vi "Fgen Basic Standard Function.vi"() -> ()   [LabVIEW 2015]
doc: "This example shows how to use Standard Function mode. This is a basic example that shows the smallest amount of code necessary to generate a standard waveform."
uses:
  <instrlib>/niFgen/niFgen.llb/niFgen Output Mode.ctl
panel:
  in  "持续时间":dbl
  in  "DC Offset":dbl format="%.4f"
  in  "Standard Waveform":u16(ring) items=["Sine", "Square", "Triangle", "Ramp Up", "Ramp Down", "DC", "Noise"]
  in  "FGEN Resource Name":refnum<k15>
  in  "Frequency":dbl=1000000.0 format="%.2p"
  in  "Amplitude":dbl=2.0 format="%0_3g"
  # "Overview: Demonstrates how to configure an NI Signal Source to generate a basic standard function.\nSoftware Requirements: NI-FGEN\nHardware Requirements: PXI-5401, PCI-5401, PXI-5402, PCI-5402, PXI-5406, PCI-5406, PXI-5411, PCI-5411, AT-5411, PXI-5412, PCI-5412, PXIe-5413, PXI-5421, PCI-5421, PXI-5422, PXIe-5423, PXI-5431, PCI-5431, PXIe-5433, PXI-5441, NI PXIe-5442, NI PXIe-5450, or NI PXIe-5451 \nInstructions:\n1. Select the FGEN Resource Name as configured in the Measurement & Automation Explorer.\n2. Select the Standard Waveform to be generated.\n3. Specify the desired Frequency for the waveform.\n4. Select to Amplitude of the waveform.\n5. Run the VI.\n6. Click Stop to stop the VI."
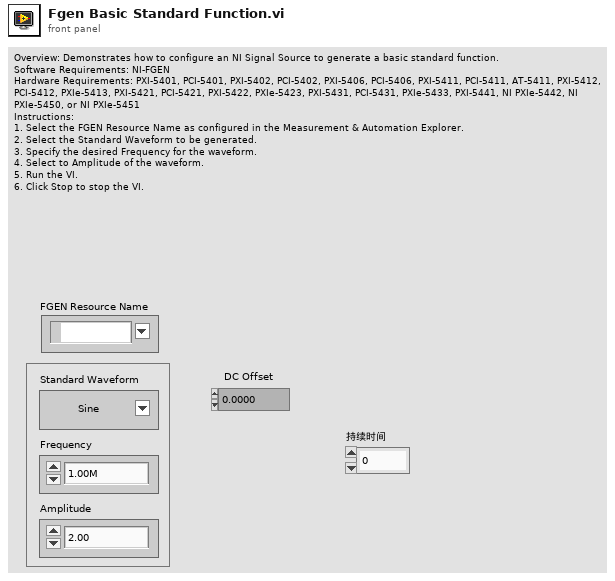
[diagram p1: front panel]
types:
  T1 = typedef "niFgen Output Mode.ctl" = u32
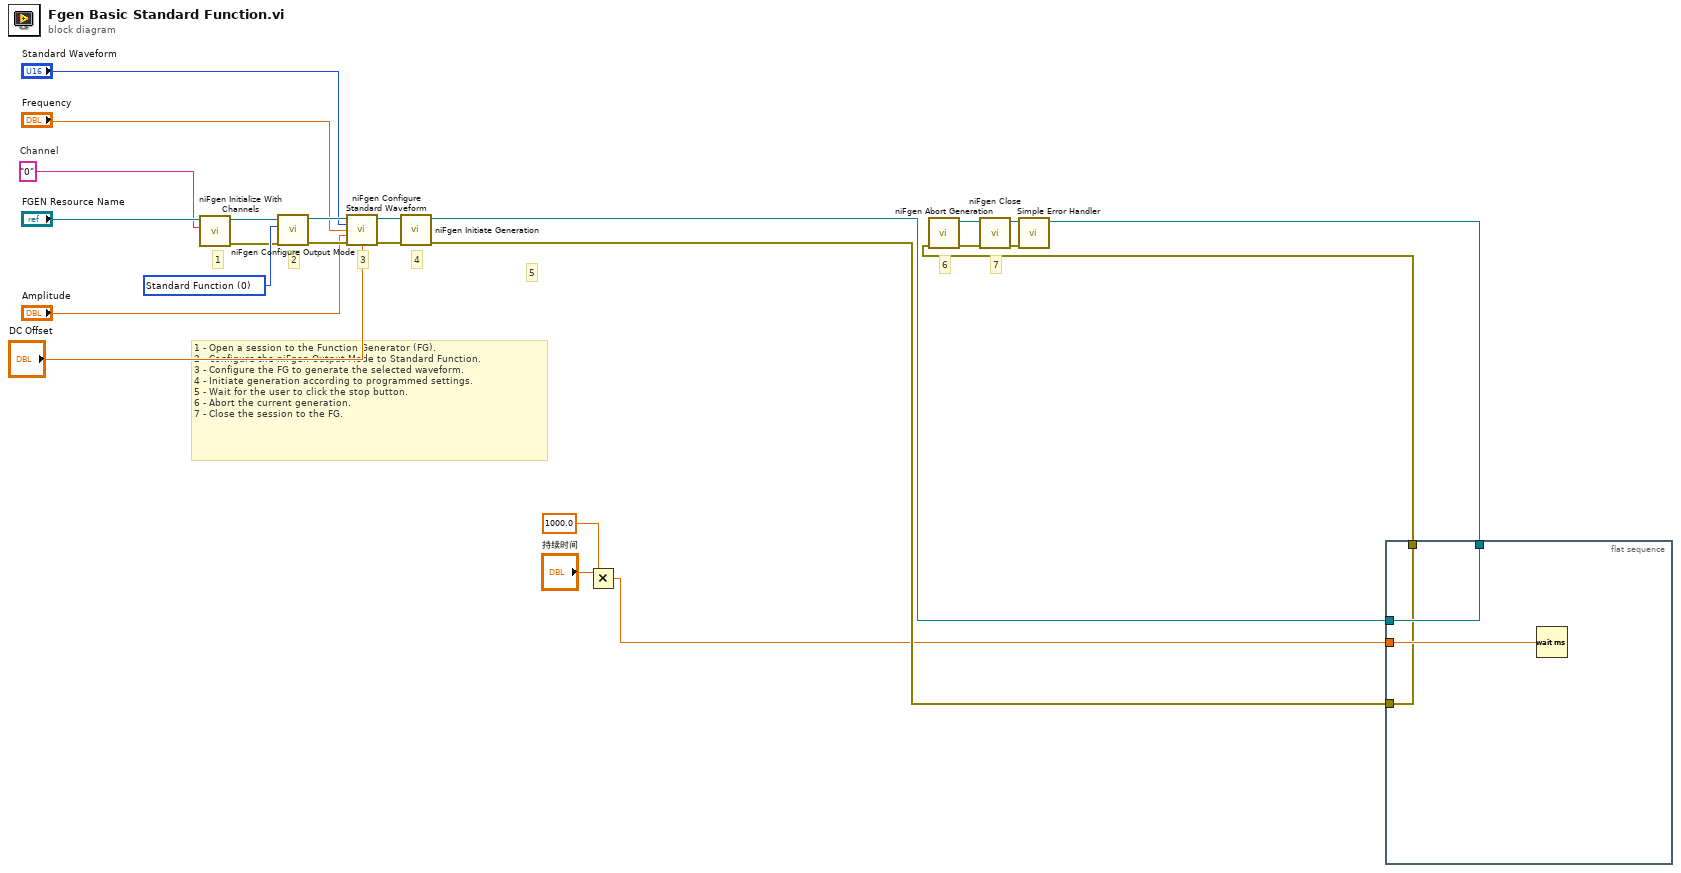
[diagram p0: block diagram]
diagram:
  w8 = "0"  # Channel
  w22 = T1 0 items=["Standard Function", "Frequency List", "Arbitrary Waveform", "Arbitrary Sequence", "Script"] ("output mode")
  # "5"
  # "7"
  # "6"
  # "4"
  # "3"
  # "2"
  # "1"
  # "1 - Open a session to the Function Generator (FG).\n2 - Configure the niFgen Output Mode to Standard Function.\n3 - Configure the FG to generate the selected waveform.\n4 - Initiate generation according to programmed settings.\n5 - Wait for the user to click the stop button.\n6 - Abort the current generation.\n7 - Close the session to the FG."
  n1 = call <instrlib>:"niFgen Initialize With Channels.vi"("Channel Name"=w8, "Resource Name"="FGEN Resource Name") -> ("error out"=w9:errorcluster, "Instrument Handle Out"=w10:refnum<k15>)  [unwired: 8 in]
  n2 = call <instrlib>:"niFgen Configure Output Mode.vi"("error in (no error)"=w9, "Output Mode (default: 0=Standard Function)"=w22, "Instrument Handle"=w10) -> ("error out"=w18:errorcluster, "Instrument Handle Out"=w19:refnum<k15>)  [unwired: 6 in]
  n3 = call <instrlib>:"niFgen Configure Standard Waveform.vi"("Instrument Handle"=w19, "Waveform"="Standard Waveform", "Frequency"="Frequency", "Amplitude"="Amplitude", "error in (no error)"=w18, "DC Offset"="DC Offset") -> ("Instrument Handle Out"=w20:refnum<k15>, "error out"=w21:errorcluster)  [unwired: 8 in]
  n4 = call <instrlib>:"niFgen Initiate Generation.vi"("error in (no error)"=w21, "Instrument Handle"=w20) -> ("error out"=w23:errorcluster, "Instrument Handle Out"=w3:refnum<k15>)  [unwired: 8 in]
  n5 = Multiply(x="持续时间", y=1000.0) -> (x*y=w4:dbl)
  n6 = call <instrlib>:"niFgen Abort Generation.vi"("error in (no error)"=w1, "Instrument Handle"=w2) -> ("error out"=w17:errorcluster, "Instrument Handle Out"=w16:refnum<k15>)  [unwired: 8 in]
  n7 = call <instrlib>:"niFgen Close.vi"("error in (no error)"=w17, "Instrument Handle"=w16) -> ("error out"=w12:errorcluster)  [unwired: 9 in]
  n8 = call <vilib>:"Simple Error Handler.vi"("error in (no error)"=w12) -> ()  [unwired: 4 in, 5 out]
  n9 = flat-sequence {
    tunnel: w4 -> [w26]
    tunnel: w3 -> [w25]
    tunnel: [w25] -> w2
    tunnel: [w24] -> w1
    tunnel: w23 -> [w24]
    frame #0 {
      n10 = Wait (ms)(milliseconds to wait=w26) -> ()  [unwired: 1 out]
    }
  }
